vi "ExecuteButtonAction.vi"(8 "ErrorIn":errorcluster, 9 "WaitForReply":bool, 10 "Command":string, 11 "ReferenceIn":refnum<class "TraceWindow.lvclass">) -> (0 "ErrorOut":errorcluster, 3 "ReferenceOut":refnum<class "TraceWindow.lvclass">)   [LabVIEW 2021, in "TraceWindow.lvlib" / "TraceWindow.lvclass"]
uses:
  TraceWindow.lvclass
  TraceWindow.lvclass/TraceWindow.ctl
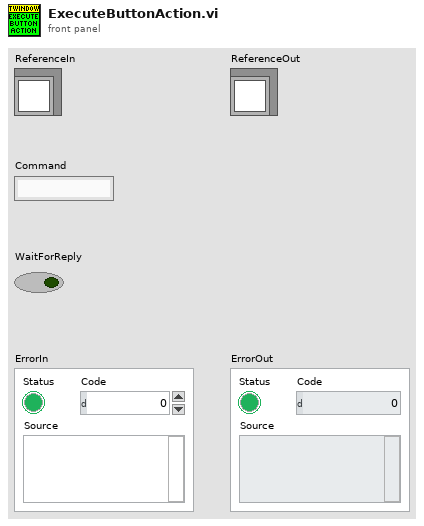
[diagram p1: front panel]
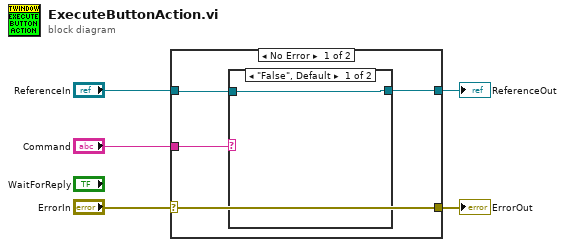
[diagram p0: block diagram]
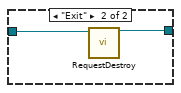
[diagram p2: hidden frame]
diagram:
  n1 = case shown="No Error" "ErrorIn" {
    selector: "ErrorIn" -> [w9 w14]
    tunnel: [w9 w14] -> w4
    tunnel: [w6 w13] -> w2
    tunnel: "ReferenceIn" -> [w7 w13]
    tunnel: "Command" -> [w8 _]
    frame No Error {
      n2 = case shown="\"False\", Default" w8 {
        tunnel: w7 -> [w10 w12]
        tunnel: [w10 w11] -> w6
        frame "False", Default {
        }
        frame "Exit" {
          n3 = call "RequestDestroy.vi"("ReferenceIn"=w12) -> ("ReferenceOut"=w11:refnum<class "TraceWindow.lvclass">)  [unwired: 9 in, 1 out]
        }
      }
    }
    frame Error {
    }
  }
  "ErrorOut" <- w4
  "ReferenceOut" <- w2
